vi "Image.vi"(2 "XRef":refnum<vi>, 3 "State In":T1) -> (0 "Image":picture)   [LabVIEW 2012, in "Unindex and Unbundle.xnode"]
doc: "This ability VI is used to describe your XNode's appearance. The origin of Image corresponds to the top-left corner of your XNode. The bounds of your XNode are used to crop this image. If you want LabVIEW to update your image, you need to inform it through the UpdateImage or UpdateImageAndBounds replies. Any areas where you do not draw are transparent, so regions intended to appear white should be explicitly drawn.\n \n Remember to localize any strings that are part of your image.\n\nDefault behavior: None.\n\nThis ability does not provide UI and OS messages are not handled."
uses:
  Unindex and Unbundle.xnode
  State.ctl
  <vilib>/picture/picture.llb/Draw True-Color Pixmap.vi
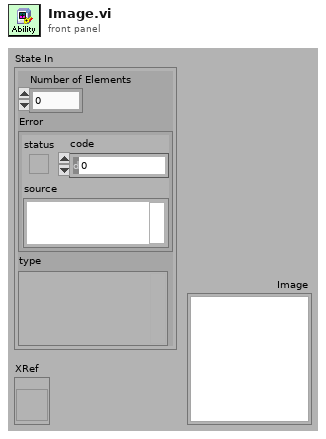
[diagram p1: front panel]
types:
  T1 = typedef "Unindex and Unbundle.xnode/State.ctl" = cluster{"Number of Elements":i32, "Error":errorcluster, "type":variant}
  T2 = typedef "imagedata.ctl" = cluster{"image type":i32, "image depth":i32, "image":u8[], "mask":u8[], "colors":u32[], "Rectangle":cluster{"left":i16, "top":i16, "right":i16, "bottom":i16}}
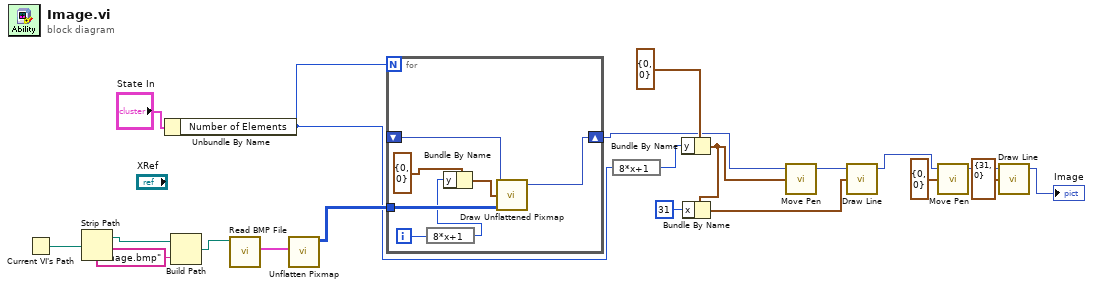
[diagram p0: block diagram]
diagram:
  n1 = Current VI's Path() -> (path=w18:path)
  n2 = Strip Path(path=w18) -> (stripped path=w19:path)  [unwired: 1 out]
  n3 = Unbundle By Name("State In") -> ("Number of Elements"=w8:i32)
  n4 = Build Path(base path=w19, name or relative path="image.bmp") -> (appended path=w16:path)
  n5 = call <vilib>:"Read BMP File.vi"("path to BMP file"=w16) -> ("image data"=w15:T2)  [unwired: 1 in, 9 out]
  n6 = call <vilib>:"Unflatten Pixmap.vi"("image data"=w15) -> ("24-bit pixmap"=w14:u32[][])  [unwired: 10 out]
  n7 = for {
    N: w8 -> [_]
    shift-right: [w21] -> w7
    shift-left: _ -> [w22]
    tunnel: w14 -> [w27]
    i -> [w26]
    n8 = expression code="8*x+1"(w26) -> (w24:i32)
    n9 = Bundle By Name(cluster=cluster{"x":i16, "y":i16} {"x"=0, "y"=0} ("top left point(0, 0)"), "y"=w24) -> (w23:cluster{"x":i16, "y":i16})
    n10 = call-poly <vilib>:"Draw Unflattened Pixmap.vi"("picture"=w22, "top left point(0, 0)"=w23, "data (RGB format)"=w27) -> ("new picture"=w21:picture)  [unwired: 1 in, 5 out]
  }
  n11 = expression code="8*x+1"(w8) -> (w9:i32)
  n12 = Bundle By Name(cluster=cluster{"x":i16, "y":i16} {"x"=0, "y"=0} ("new position"), "y"=w9) -> (w6:cluster{"x":i16, "y":i16})
  n13 = Bundle By Name(cluster=w6, "x"=i16 31 ("y")) -> (w4:cluster{"x":i16, "y":i16})
  n14 = call <vilib>:"Move Pen.vi"("new position"=w6, "picture"=w7) -> ("new picture"=w11:picture)  [unwired: 1 in, 2 out]
  n15 = call <vilib>:"Draw Line.vi"("picture"=w11, "end point"=w4) -> ("new picture"=w3:picture)  [unwired: 3 in, 4 out]
  n16 = call <vilib>:"Move Pen.vi"("new position"=cluster{"x":i16, "y":i16} {"x"=0, "y"=0}, "picture"=w3) -> ("new picture"=w13:picture)  [unwired: 1 in, 2 out]
  n17 = call <vilib>:"Draw Line.vi"("picture"=w13, "end point"=cluster{"x":i16, "y":i16} {"x"=31, "y"=0}) -> ("new picture"=→"Image":picture)  [unwired: 3 in, 4 out]
